vi "TEST Control Value To Registry (Prepend).vi"() -> ()   [LabVIEW 2013, in "Carya Config.lvclass"]
doc: "Copyright 2018, Carya Automatisering, Wiebe Walstra."
uses:
  Carya Config.lvclass
  CConfig Ctrl Ref Accessor/Registry Ctrl Ref Accessor.lvclass
  CConfig Variant Accessor/CConfig Variant Accessor.lvclass
panel:
  out "data":T1
  out "error out":errorcluster
  out "String":string
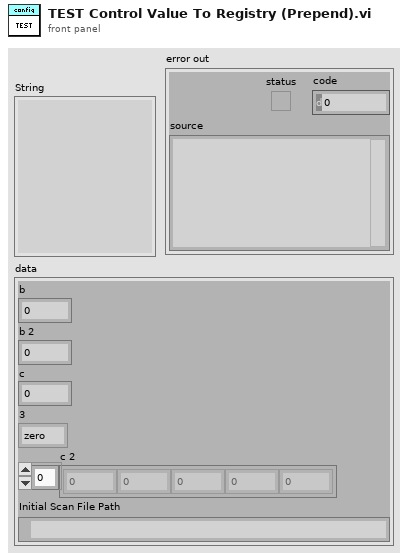
[diagram p1: front panel]
types:
  T1 = cluster{"b":i32, "b 2":i32, "c":csg, "3":enum16{"zero", "one", "two"}, "c 2":sgl[], "Initial Scan File Path":path}
  T2 = cluster{"q":i32[], cluster{"b":i32, "b 2":i32, "c":csg, "3":enum16{"zero", "one", "two"}, "c 2":sgl[], "Initial Scan File Path":path}}
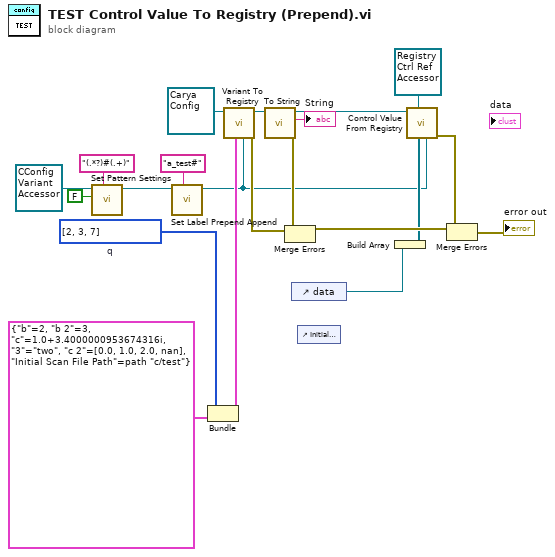
[diagram p0: block diagram]
diagram:
  w12 = i32[] [2, 3, 7]  # q
  n1 = call "Set Pattern Settings.vi"("Pattern [section_key]"="(.*?)#(.+)", "Swap match [F]"=FALSE, "CConfig Variant Accessor in"=refnum<class "CConfig Variant Accessor.lvclass"> refnum) -> ("CConfig Variant Accessor out"=w3:refnum<class "CConfig Variant Accessor.lvclass">)  [unwired: 7 in, 1 out]
  n2 = call "Set Label Prepend Append.vi"("Label Prepend"="a_test#", "CConfig Variant Accessor in"=w3) -> ("CConfig Variant Accessor out"=w4:refnum<class "CConfig Variant Accessor.lvclass">)  [unwired: 8 in, 1 out]
  n3 = Bundle("q"=w12, T1 {"b"=2, "b 2"=3, "c"=1.0+3.4i, "3"=enum."two", "c 2"=[0.0, 1.0, 2.0, nan], "Initial Scan File Path"=path "c:/test"}) -> (w14:T2)  [unwired: 1 in]
  n4 = call "Variant To Registry.vi"("Registry Variant Accessor in"=w4, "Variant"=w14, "Carya Config in"=refnum<class "Carya Config.lvclass"> refnum) -> ("error out"=w17:errorcluster, "Carya Config out"=w20:refnum<class "Carya Config.lvclass">)  [unwired: 5 in, 2 out]
  n5 = call-dynamic "To String.vi"("Carya Config in"=w20) -> ("error out"=w18:errorcluster, "String"=→"String":string, "Carya Config out"=w10:refnum<class "Carya Config.lvclass">)  [unwired: 8 in]
  n6 = Merge Errors(w17, w18) -> (w16:errorcluster)
  n7 = control-ref of="data"() -> (w7:refnum<vi>)
  n8 = control-ref of="Initial Scan File Path"() -> ()  [unwired: 1 out]
  n9 = Build Array(w7) -> (w9:refnum<vi>[])
  n10 = call "Control Value From Registry.vi"("Registry Variant Accessor (optional)"=w4, "Controls"=w9, "Registry Control Reference Accessor (optional)"=refnum<class "Registry Ctrl Ref Accessor.lvclass"> refnum ("Registry Control Reference Accessor.lvclass"), "Registry Object in"=w10) -> ("error out"=w8:errorcluster)  [unwired: 5 in, 2 out]
  n11 = Merge Errors(w16, w8) -> (→"error out":errorcluster)
